vi "Read Numeric.vi"(8 "error in (no error)":errorcluster, 11 "myClassWOPropFolder in":refnum<class "myClassWOPropFolder.lvclass">) -> (0 "error out":errorcluster, 2 "Numeric":dbl, 3 "myClassWOPropFolder out":refnum<class "myClassWOPropFolder.lvclass">)   [LabVIEW 2017, in "myClassWOPropFolder.lvclass"]
uses:
  myClassWOPropFolder.lvclass
  myClassWOPropFolder.lvclass/myClassWOPropFolder.ctl
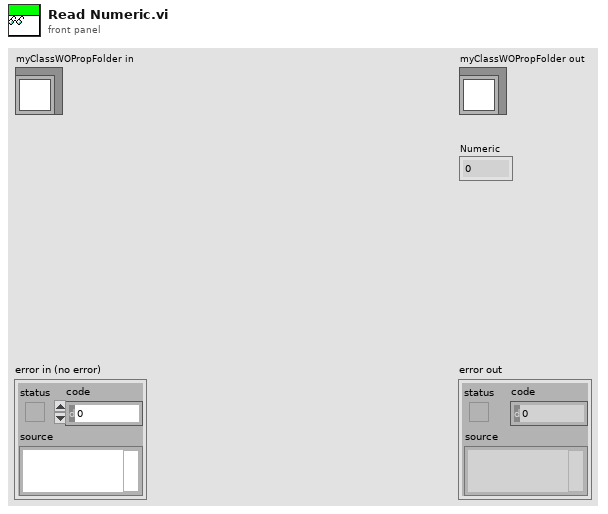
[diagram p1: front panel]
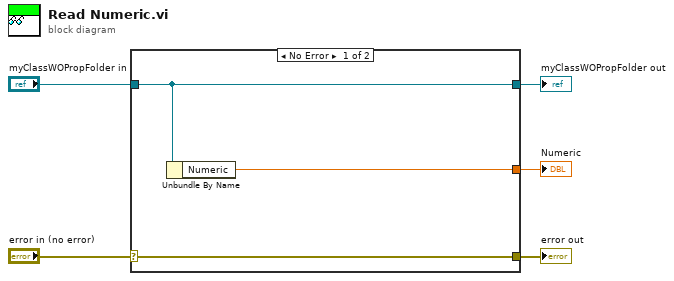
[diagram p0: block diagram]
diagram:
  n1 = case shown="No Error" "error in (no error)" {
    selector: "error in (no error)" -> [w8 w9]
    tunnel: [w8 w9] -> w4
    tunnel: [w7 w10] -> w2
    tunnel: "myClassWOPropFolder in" -> [w7 w10]
    tunnel: [w6 _] -> w1
    frame No Error {
      n2 = Unbundle By Name(w7) -> ("Numeric"=w6:dbl)
    }
    frame Error {
    }
  }
  "error out" <- w4
  "myClassWOPropFolder out" <- w2
  "Numeric" <- w1
